vi "Close.vi"(8 "error in (no error)":errorcluster) -> (0 "error out":errorcluster)   [LabVIEW 2017, in "Drive Train.lvlib"]
uses:
  Drive Train.lvlib
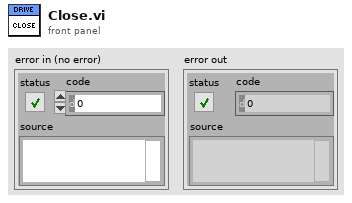
[diagram p1: front panel]
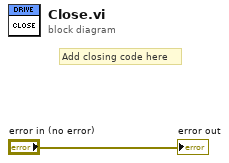
[diagram p0: block diagram]
diagram:
  # "Add closing code here"
  "error out" <- "error in (no error)"
